vi "example_hmi_get_references.vi"(8 "error in (no error)":errorcluster, 10 "control_search []":string[](array[string]), 11 "vi_reference":refnum<vi>) -> (0 "error out":errorcluster, 3 "references":cluster{refnum<vi>[]}[](array[cluster]))   [LabVIEW 2015, in "lv-pagination.lvlib"]
doc: "This is used by example 2 to grab all of the references within the provided VI reference to get all the references that match the control search."
uses:
  lv-pagination.lvlib
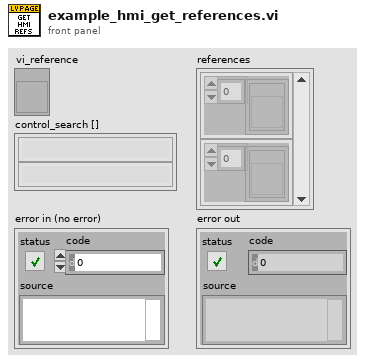
[diagram p1: front panel]
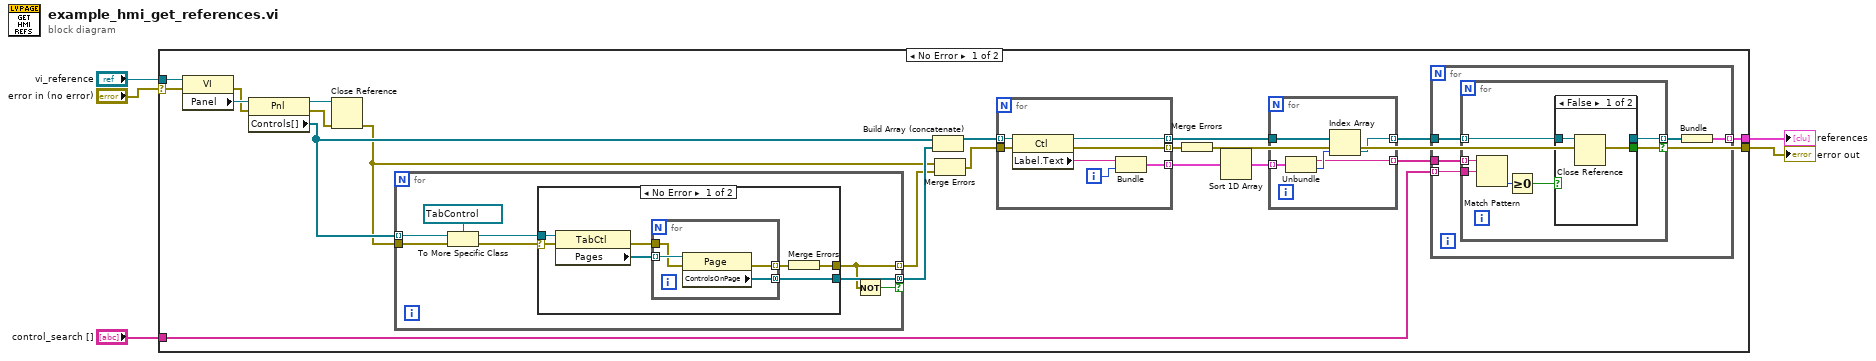
[diagram p0: block diagram]
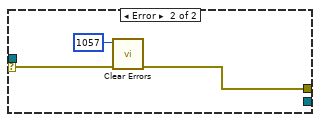
[diagram p2: hidden frame]
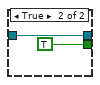
[diagram p3: hidden frame]
diagram:
  n1 = case shown="No Error" "error in (no error)" {
    selector: "error in (no error)" -> [w17 w76]
    tunnel: [w6 w76] -> w5
    tunnel: "vi_reference" -> [w18 _]
    tunnel: [w16 _] -> w1
    tunnel: "control_search []" -> [w15 _]
    frame No Error {
      n2 = property class="VI"(reference=w18, error in=w17) -> (error out=w23:errorcluster, "Panel"=w26:refnum<vi>)  [unwired: 1 out]
      n3 = property class="Pnl"(reference=w26, error in=w23) -> (reference out=w25:refnum<vi>, error out=w24:errorcluster, "Controls[]"=w22:refnum<vi>[])
      n4 = Close Reference(reference=w25, error in (no error)=w24) -> (error out=w19:errorcluster)
      n5 = for {
        tunnel: w22 -> [w41] mode=indexing
        tunnel: [w37] -> w21 mode=concatenating if=w36
        tunnel: w19 -> [w35]
        tunnel: [w34] -> w20 mode=indexing
        n6 = To More Specific Class(target class=refnum<vi> refnum ("tab_control"), reference=w41, error in=w35) -> (specific class reference=w38:refnum<vi>, error out=w39:errorcluster)
        n7 = case shown="No Error" w39 {
          selector: w39 -> [w48 w55]
          tunnel: w38 -> [w47 _]
          tunnel: [w45 _] -> w37
          tunnel: [w42 w54] -> w34
          frame No Error {
            n8 = property class="TabCtl"(reference=w47, error in=w48) -> (error out=w44:errorcluster, "Pages"=w46:refnum<vi>[])  [unwired: 1 out]
            n9 = for {
              tunnel: w46 -> [w52] mode=indexing
              tunnel: [w51] -> w45 mode=concatenating
              tunnel: w44 -> [w50]
              tunnel: [w49] -> w43 mode=indexing
              n10 = property class="Page"(reference=w52, error in=w50) -> (error out=w49:errorcluster, "ControlsOnPage"=w51:refnum<vi>[])  [unwired: 1 out]
            }
            n11 = Merge Errors(w43) -> (w42:errorcluster)
          }
          frame Error {
            n12 = call <vilib>:"Clear Errors.vi"("error in (no error)"=w55, "specific error code to clear (0: all)"=1057) -> ("error out"=w54:errorcluster)  [unwired: 4 in, 1 out]
          }
        }
        n13 = Not(x=w34) -> (.not. x?=w36:bool)
      }
      n14 = Build Array (concatenate)(w22, w21) -> (w14:refnum<vi>[])
      n15 = Merge Errors(w19, w20) -> (w13:errorcluster)
      n16 = for {
        tunnel: w14 -> [w33] mode=indexing
        tunnel: w13 -> [w31]
        tunnel: [w32] -> w11 mode=indexing
        tunnel: [w30] -> w9 mode=indexing
        tunnel: [w28] -> w12 mode=indexing
        i -> [w29]
        n17 = property class="Ctl"(reference=w33, error in=w31) -> (reference out=w32:refnum<vi>, error out=w30:errorcluster, "Label.Text"=w27:string)
        n18 = Bundle("Label.Text"=w27, w29) -> (w28:cluster{"Label.Text":string, i32})  [unwired: 1 in]
      }
      n19 = Merge Errors(w9) -> (w6:errorcluster)
      n20 = Sort 1D Array(array=w12) -> (sorted array=w10:cluster{"Label.Text":string, i32}[])
      n21 = for {
        tunnel: w11 -> [w60]
        tunnel: w10 -> [w59] mode=indexing
        tunnel: [w57] -> w7 mode=indexing
        tunnel: [w56] -> w8 mode=indexing
        n22 = Unbundle(w59) -> ("Label.Text"=w57:string, w58:i32)
        n23 = Index Array(array=w60, index=w58) -> (element=w56:refnum<vi>)
      }
      n24 = for {
        tunnel: w8 -> [w65]
        tunnel: [w63] -> w16 mode=indexing
        tunnel: w15 -> [w62] mode=indexing
        tunnel: w7 -> [w61]
        n25 = for {
          tunnel: w65 -> [w71] mode=indexing
          tunnel: [w70] -> w64 mode=indexing if=w69
          tunnel: w62 -> [w66]
          tunnel: w61 -> [w67] mode=indexing
          n26 = Match Pattern(string=w67, regular expression=w66) -> (offset past match=w68:i32)  [unwired: 1 in, 3 out]
          n27 = Greater Or Equal To 0?(x=w68) -> (x >= 0?=w72:bool)
          n28 = case shown="False" w72 {
            tunnel: w71 -> [w73 w75]
            tunnel: [_ w75] -> w70
            tunnel: [_ TRUE] -> w69
            frame False {
              n29 = Close Reference(reference=w73) -> ()  [unwired: 1 in, 1 out]
            }
            frame True {
            }
          }
        }
        n30 = Bundle(w64) -> (w63:cluster{refnum<vi>[]})  [unwired: 1 in]
      }
    }
    frame Error {
    }
  }
  "error out" <- w5
  "references" <- w1
